vi "color.vi"() -> ()   [LabVIEW 2014]
uses:
  <vilib>/myRIO/Instrument Drivers/Onboard IO/DI Block/vis/Read.vi
  <vilib>/myRIO/Common/Instrument Driver Framework/myRIO v1.0/UART/vis/myRIO v1.0 Close UART.vi
  <vilib>/myRIO/Instrument Drivers/Onboard IO/DI Block/vis/Smart Open.vi
  <vilib>/Utility/error.llb/Error Cluster From Error Code.vi
  <vilib>/myRIO/Common/Instrument Driver Framework/myRIO v1.0/DI Block/vis/myRIO v1.0 DI Block Read.vi
  <vilib>/myRIO/Common/Instrument Driver Framework/Utilities/vis/FPGA Ref Manager.vi
  <vilib>/myRIO/Common/Instrument Driver Framework/myRIO v1.0/myRIO v1.0 Reset FPGA.vi
  <vilib>/myRIO/Common/Instrument Driver Framework/myRIO v1.0/IRQ/vis/myRIO v1.0 IRQ Info FGV.vi
  <vilib>/myRIO/Common/Instrument Driver Framework/myRIO v1.0/IRQ/vis/myRIO v1.0 Timer IRQ Info FGV.vi
  <vilib>/myRIO/Common/Instrument Driver Framework/myRIO v1.0/IRQ/vis/myRIO v1.0 ISR Agent.vi
  <vilib>/measure/matone.llb/Extract Single Tone Information 1 Chan.vi
  <vilib>/myRIO/Instrument Drivers/Utilities/Utilities.lvlib
  <vilib>/measure/NI_MAPro.lvlib
panel:
  out "A/DI0 (N Samples) (Pin 11)":bool[](array[boolean])
  in  "s1":bool
  in  "STOP":bool
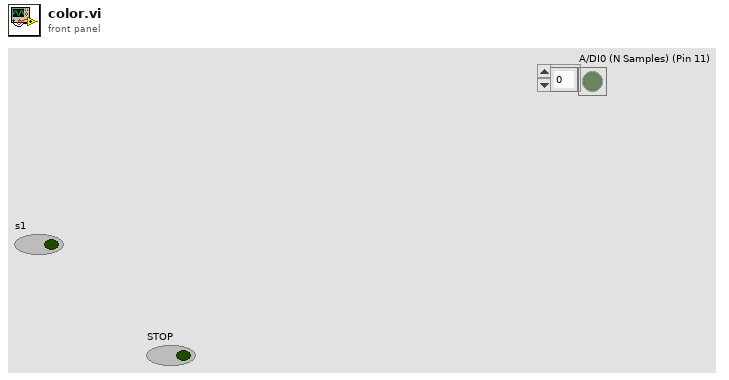
[diagram p1: front panel]
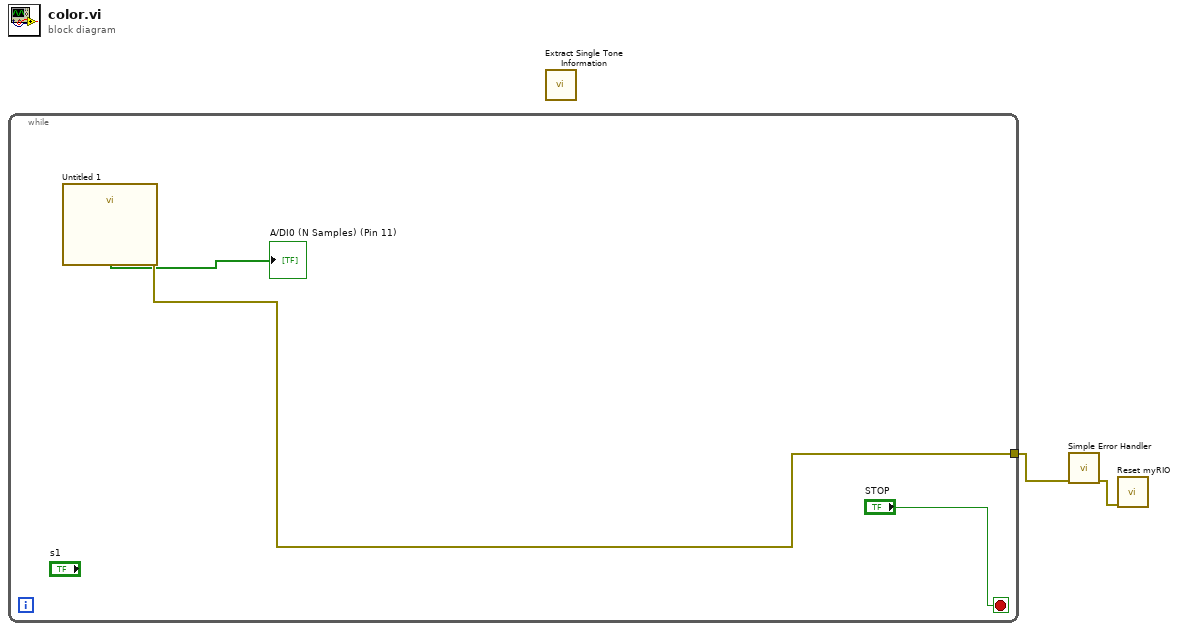
[diagram p0: block diagram]
diagram:
  n1 = while {
    tunnel: [w4] -> w1
    stop <- "STOP" stop-if-true
    n2 = call "Untitled 1.vi"() -> ("A/DI0 (N Samples) (Pin 11)"=→"A/DI0 (N Samples) (Pin 11)":bool[], "error out"=w4:errorcluster)  [unwired: 26 in]
  }
  n3 = call-poly <vilib>:"Extract Single Tone Information.vi"() -> ()  [unwired: 6 in, 6 out]
  n4 = call <vilib>:"Simple Error Handler.vi"("error in (no error)"=w1) -> ("error out"=w2:errorcluster)  [unwired: 4 in, 4 out]
  n5 = call <vilib>:"Reset myRIO.vi"("error in (no error)"=w2) -> ()  [unwired: 10 in, 1 out]
